vi "Pre Launch Init.vi"(11 "UDP_transmitter in":refnum<class "UDP_transmitter.lvclass">) -> (0 "error out":errorcluster, 3 "UDP_transmitter out":refnum<class "UDP_transmitter.lvclass">)   [LabVIEW 2025, in "UDP_transmitter.lvlib" / "UDP_transmitter.lvclass"]
doc: "(<B>Filename</B>: Actor Framework.lvlib:Actor.lvclass:Pre Launch Init.vi)\n\nDefines behavior that occurs after the Launch Nested Actor method is invoked but before the actor's Actor Core method begins running.\n\nBy default, this method does nothing. A descendant class may override it to define behavior."
uses:
  UDP_transmitter.lvclass
  UDP_transmitter.lvclass/UDP_transmitter.ctl
  <vilib>/ActorFramework/Actor/Actor.lvclass
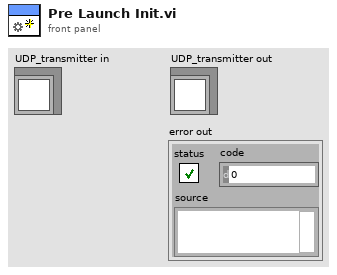
[diagram p1: front panel]
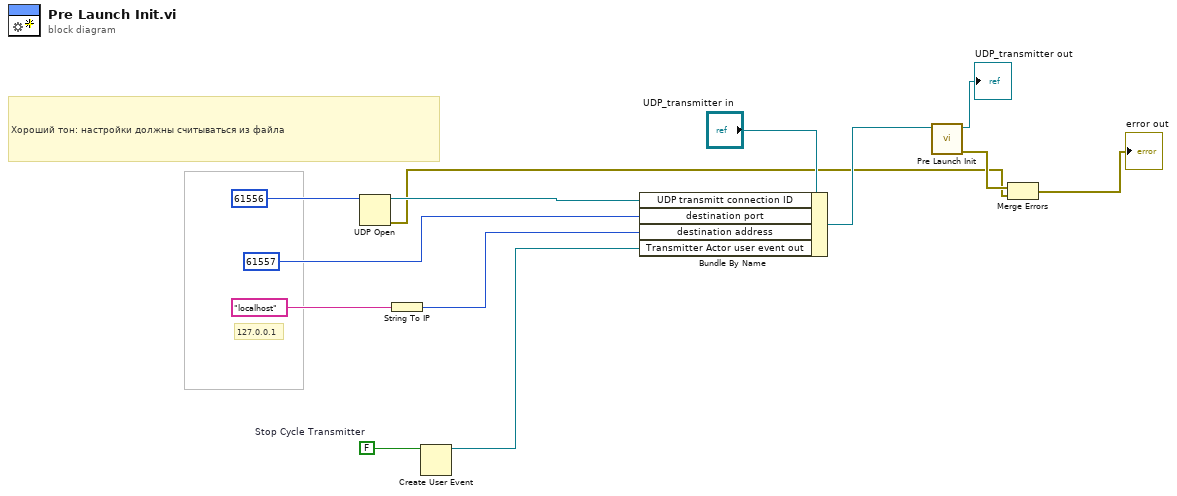
[diagram p0: block diagram]
diagram:
  w2 = FALSE  # Stop Cycle Transmitter
  # "Хороший тон: настройки должны считываться из файла"
  # "127.0.0.1"
  n1 = UDP Open(11:u16 61556 ("port")) -> (port=w10:refnum<k16>, 0:w6:errorcluster)  [unwired: 4 in, 1 out]
  n2 = String To IP(1:"localhost" ("name")) -> (0:w3:u32)
  n3 = Create User Event(user event datatype=w2) -> (user event=w1:refnum<user-event>)  [unwired: 1 in, 1 out]
  n4 = Bundle By Name(cluster="UDP_transmitter in", "UDP transmitt connection ID"=w10, "destination port"=u16 61557 ("port or service name"), "destination address"=w3, "Transmitter Actor user event out"=w1) -> (w8:refnum<class "UDP_transmitter.lvclass">)
  n5 = call-parent "Pre Launch Init.vi"("Actor in"=w8) -> ("error out"=w7:errorcluster, "Actor out"=→"UDP_transmitter out":refnum<class "UDP_transmitter.lvclass">)  [unwired: 9 in]
  n6 = Merge Errors(w7, w6) -> (→"error out":errorcluster)
